vi "Get BLISS_Custom Error.vi"(8 "error in (no error)":errorcluster, 9 "search criteria":string, 10 "Array":path[](array[path]), 11 "Parent path":path) -> (0 "error out":errorcluster)   [LabVIEW 2020]
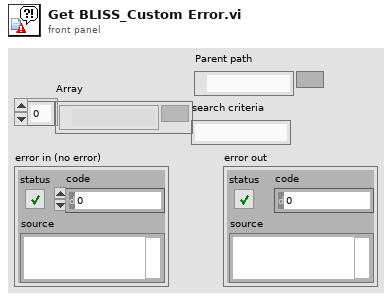
[diagram p1: front panel]
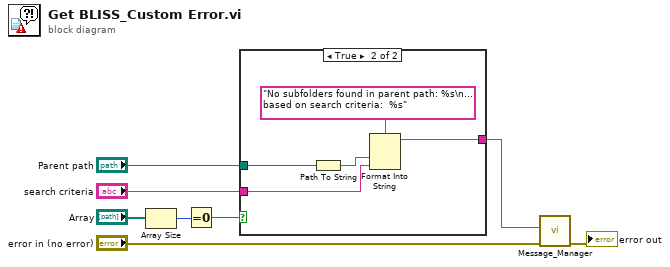
[diagram p0: block diagram]
diagram:
  n1 = Array Size(array="Array") -> (size(s)=w8:i32)
  n2 = Equal To 0?(x=w8) -> (x = 0?=w2:bool)
  n3 = case shown="True" w2 {
    tunnel: "Parent path" -> [_ w13]
    tunnel: "search criteria" -> [_ w11]
    tunnel: [_ w9] -> w1
    frame False {
    }
    frame True {
      n4 = Path To String(path=w13) -> (string=w10:string)
      n5 = Format Into String(format string="No subfolders found in parent path: %s\n... based on search criteria:  %s", w10, w11) -> (resulting string=w9:string)  [unwired: 2 in, 1 out]
    }
  }
  n6 = call "Message_Manager.vi"("error in"="error in (no error)", "New Entry"=w1) -> ("error out"=→"error out":errorcluster)  [unwired: 4 in, 5 out]
